vi "RSZVB Define Mixer Delay Receiver.vi"(8 "error in (no error)":errorcluster {"code" format="%.0x"}, 9 "Measurement Setup (\"192.168.0.1\")":string="192.168.0.1", 11 "VISA session":refnum<visa-resource-name>) -> (0 "error out":errorcluster {"code" format="%.0x"}, 3 "dup VISA session":refnum<visa-resource-name>)   [LabVIEW 2011]
doc: "Configures a network analyzer as an external receiver for the mixer delay measurement and adds it to the list of available receivers. \n\nNotes:\n\n(1) This mode requires options R&S ZVA-K9 and R&S ZVA-K4\n\nRemote-control command(s):\nSYSTem:COMMunicate:RDEVice:RECeiver:DEFine"
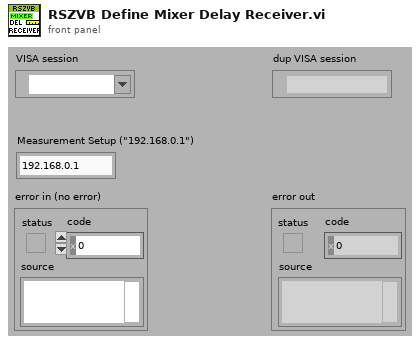
[diagram p1: front panel]
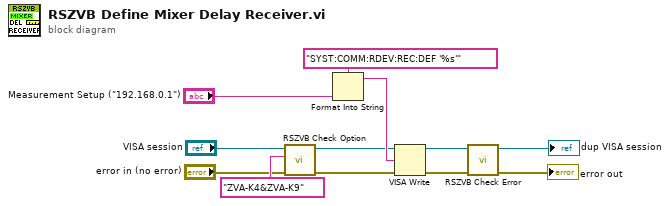
[diagram p0: block diagram]
diagram:
  n1 = call "RSZVB Check Option.vi"("error in (no error)"="error in (no error)", "Options"="ZVA-K4&ZVA-K9", "VISA session"="VISA session") -> ("error out"=w3:errorcluster, "dup VISA session"=w4:refnum<visa-resource-name>)  [unwired: 7 in]
  n2 = Format Into String(format string="SYST:COMM:RDEV:REC:DEF '%s'", "Measurement Setup (\"192.168.0.1\")") -> (resulting string=w9:string)  [unwired: 2 in, 1 out]
  n3 = VISA Write(VISA resource name=w4, write buffer=w9, error in (no error)=w3) -> (VISA resource name out=w11:refnum<visa-resource-name>, error out=w12:errorcluster)  [unwired: 1 out]
  n4 = call "RSZVB Check Error.vi"("error in (no error)"=w12, "VISA session"=w11) -> ("error out"=→"error out":errorcluster, "dup VISA session"=→"dup VISA session":refnum<visa-resource-name>)  [unwired: 8 in]
